vi "BRig_FPGA_resetOutputs_PortA.vi"   [LabVIEW 2014]
uses:
  <vilib>/rvi/eio/common/nirviEmuTemplateMethod_errors.vi
  <vilib>/eio/EIONode/EIONode.xnode
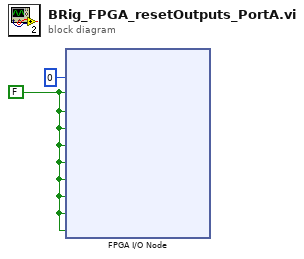
[diagram p0: block diagram]
diagram:
  w1 = FALSE ("ConnectorA/DIO3")
  n1 = xnode "FPGA I/O Node"("ConnectorB/AO0"=u16 0 ("ConnectorA/AO0"), "ConnectorA/DIO0"=w1, "ConnectorA/DIO1"=w1, "ConnectorA/DIO2"=w1, "ConnectorA/DIO3"=w1, "ConnectorA/DIO4"=w1, "ConnectorA/DIO5"=w1, "ConnectorA/DIO6"=w1, "ConnectorA/DIO7"=w1, "ConnectorA/DIO14"=w1) -> ()  [unwired: 10 in, 10 out]
